vi "Deinitialize.vi"(8 "error in":errorcluster, 11 "connection reference":T1) -> (0 "error out":errorcluster)   [LabVIEW 2023, in "SQL Database.lvlib"]
uses:
  SQL Database.lvlib
  <vilib>/addons/database/NI_Database_API.lvlib
  <vilib>/addons/database/Connection.llb/Conn ObjectReference.ctl
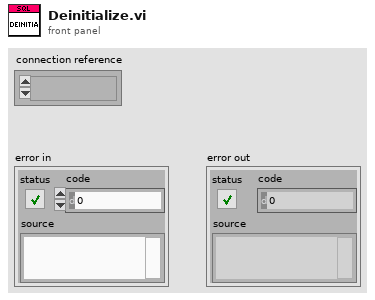
[diagram p1: front panel]
types:
  T1 = typedef "NI_Database_API.lvlib/Conn ObjectReference.ctl" = refnum<k1>
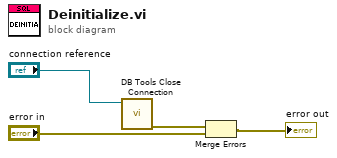
[diagram p0: block diagram]
diagram:
  n1 = call <vilib>:"DB Tools Close Connection.vi"("connection reference"="connection reference") -> ("error out"=w3:errorcluster)  [unwired: 6 in]
  n2 = Merge Errors(w3, "error in") -> (→"error out":errorcluster)
